vi "Worksheet DOE Audit.vi"(5 "Write Form":bool, 6 "Add?":bool, 7 "Calibration Data":string[][](array[string]), 8 "Low Power\nSwitch":bool, 9 "DOE Data":T1={"Technician"="", "Date"="", "Model"="", "Serial"="", "Total Dry Time(m)"=0.0, "Bone Dry Wt"=0.0, "Initial Wt"=0.0, "Final Wt"=0.0, "Initial Ret"=0.0, "Final Ret"=0.0, "Elect Energy Used"=0.0, "Gas Meter Temp"=0.0, "Gas Meter Pres"=0.0, "Gas Volume"=0.0, "Barometer Temp"=70.0, "Barometer Pres"=0.0, "Gas Corr Fact"=0.0, "Cor Gas Vol"=0.0, "Gas Heat Val"=0.0, "Gas Energy BTU"=0.0, "Gas Energy kwh 4%"=0.0, "Elect Energy kwh 4%"=0.0, "Total  Energy 4%"=0.0, "Gas Vol Init"=0.0, "Gas Vol Fin"=0.0, "Start Time(s)"=0.0, "End Time(s)"=0.0, "Elect Energy Start"=0.0, "Elect Energy End"=0.0, "Per Cycle Efficency"=0.0, "Annual Consumption"=0.0, "Load Cycles"="", "Ambinet Temp"="", "Ambinet RH"="", "Per Cycle Off Mode/Standby Power"=0.0, "Total Energy (Gas + Elect)"=0.0, "Combined Energy Factor"=0.0, "Off Mode Power"=0.0, "Exhaust"="", "Washer Water Temperature ( 60 ± 5°F )"="", "Supply Voltage"="", "Reference Temperature (F)"="", "Reference Pressure (psi)"="", "Standby Power"=0.0}, 10 "2015?":bool) -> (0 "String":string, 1 "2015 array":string[][](array[string]), 2 "DOE Data Out":T1={"Technician"="", "Date"="", "Model"="", "Serial"="", "Total Dry Time(m)"=0.0, "Bone Dry Wt"=0.0, "Initial Wt"=0.0, "Final Wt"=0.0, "Initial Ret"=0.0, "Final Ret"=0.0, "Elect Energy Used"=0.0, "Gas Meter Temp"=0.0, "Gas Meter Pres"=0.0, "Gas Volume"=0.0, "Barometer Temp"=70.0, "Barometer Pres"=0.0, "Gas Corr Fact"=0.0, "Cor Gas Vol"=0.0, "Gas Heat Val"=0.0, "Gas Energy BTU"=0.0, "Gas Energy kwh 4%"=0.0, "Elect Energy kwh 4%"=0.0, "Total  Energy 4%"=0.0, "Gas Vol Init"=0.0, "Gas Vol Fin"=0.0, "Start Time(s)"=0.0, "End Time(s)"=0.0, "Elect Energy Start"=0.0, "Elect Energy End"=0.0, "Per Cycle Efficency"=0.0, "Annual Consumption"=0.0, "Load Cycles"="", "Ambinet Temp"="", "Ambinet RH"="", "Per Cycle Off Mode/Standby Power"=0.0, "Total Energy (Gas + Elect)"=0.0, "Combined Energy Factor"=0.0, "Off Mode Power"=0.0, "Exhaust"="", "Washer Water Temperature ( 60 ± 5°F )"="", "Supply Voltage"="", "Reference Temperature (F)"="", "Reference Pressure (psi)"="", "Standby Power"=0.0})   [LabVIEW 2012]
uses:
  DOE Audit Data.ctl
panel:
  out "Array":string[](array[string])=["tech", "mod", "sn", "loadcy", "dat", "exh", "baro", "wwt", "gm", "sc", "wt5", "gmpt", "ni", "barop", "barot", "rhs", "rhs2", "ts1", "ts2", "gtt", "sca", "tp1", "tp2", "ambt", "ambrh", "gmp", "gmt", "sv", "ghv", "rp", "rt", "bdw", "iw", "fw", "iret", "fr", "tdt", "eeu", "gv", "gcf", "gebtu", "tege", "te4", "om", "sp", "pcomsp", "P", "cef", "ac"]
  out "Column Data":string[](array[string])
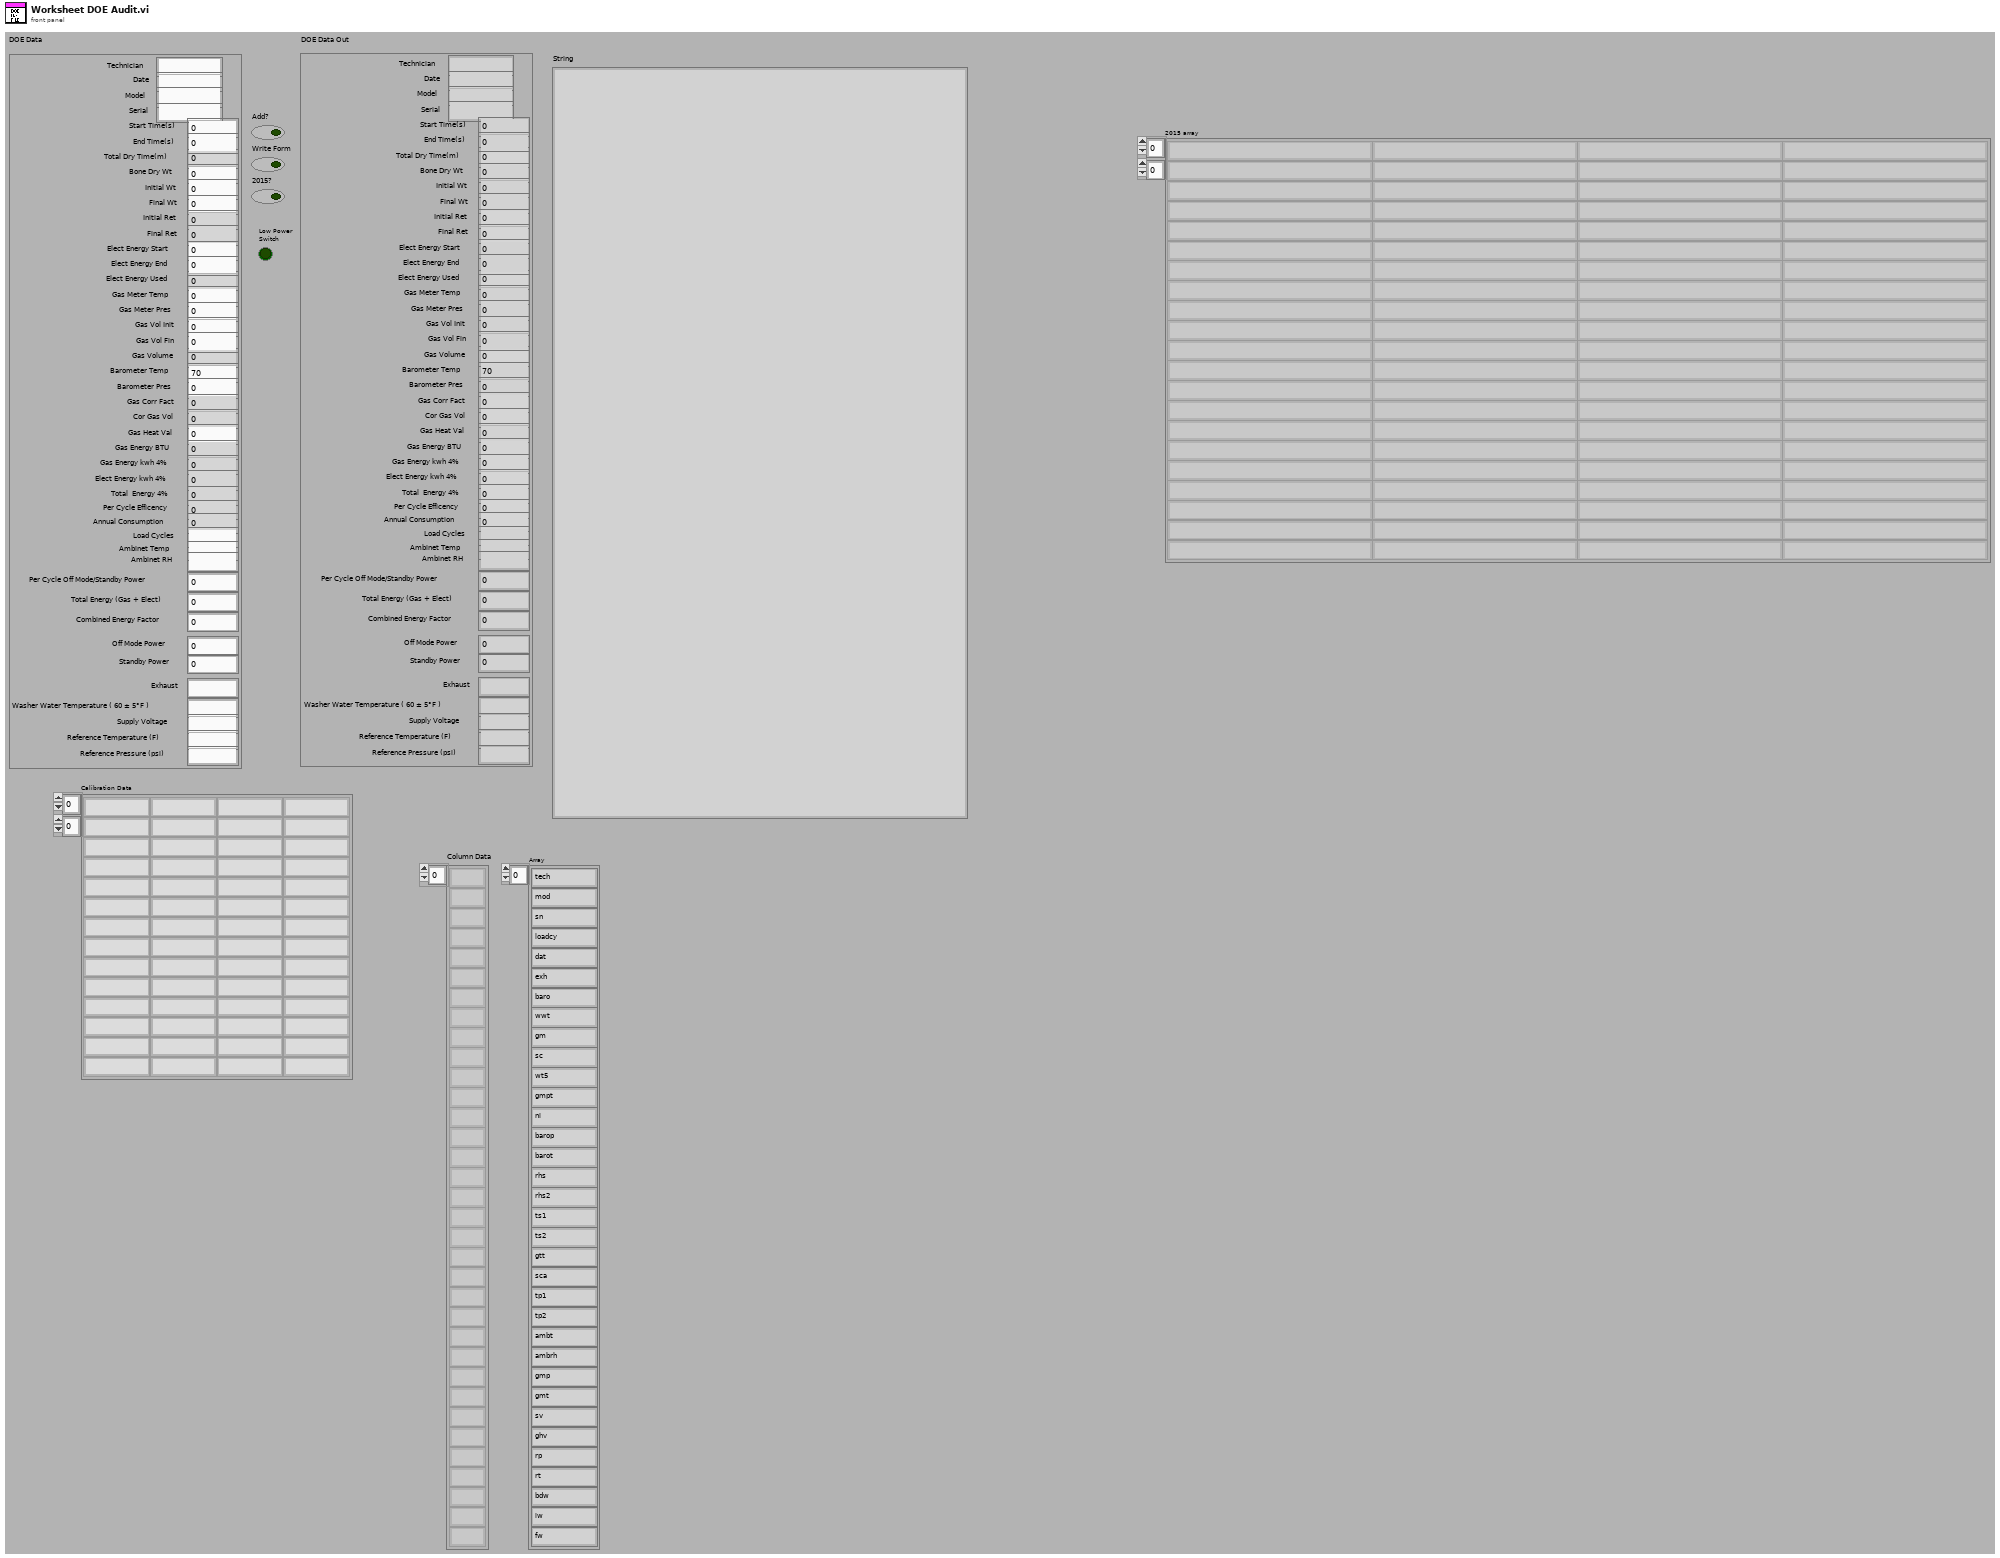
[diagram p1: front panel]
types:
  T1 = typedef "DOE Audit Data.ctl" = cluster{"Technician":string, "Date":string, "Model":string, "Serial":string, "Total Dry Time(m)":dbl, "Bone Dry Wt":dbl, "Initial Wt":dbl, "Final Wt":dbl, "Initial Ret":dbl, "Final Ret":dbl, "Elect Energy Used":dbl, "Gas Meter Temp":dbl, "Gas Meter Pres":dbl, "Gas Volume":dbl, "Barometer Temp":dbl, "Barometer Pres":dbl, "Gas Corr Fact":dbl, "Cor Gas Vol":dbl, "Gas Heat Val":dbl, "Gas Energy BTU":dbl, "Gas Energy kwh 4%":dbl, "Elect Energy kwh 4%":dbl, "Total  Energy 4%":dbl, "Gas Vol Init":dbl, "Gas Vol Fin":dbl, "Start Time(s)":dbl, "End Time(s)":dbl, "Elect Energy Start":dbl, "Elect Energy End":dbl, "Per Cycle Efficency":dbl, "Annual Consumption":dbl, "Load Cycles":string, "Ambinet Temp":string, "Ambinet RH":string, "Per Cycle Off Mode/Standby Power":dbl, "Total Energy (Gas + Elect)":dbl, "Combined Energy Factor":dbl, "Off Mode Power":dbl, "Exhaust":string, "Washer Water Temperature ( 60 ± 5°F )":string, "Supply Voltage":string, "Reference Temperature (F)":string, "Reference Pressure (psi)":string, "Standby Power":dbl}
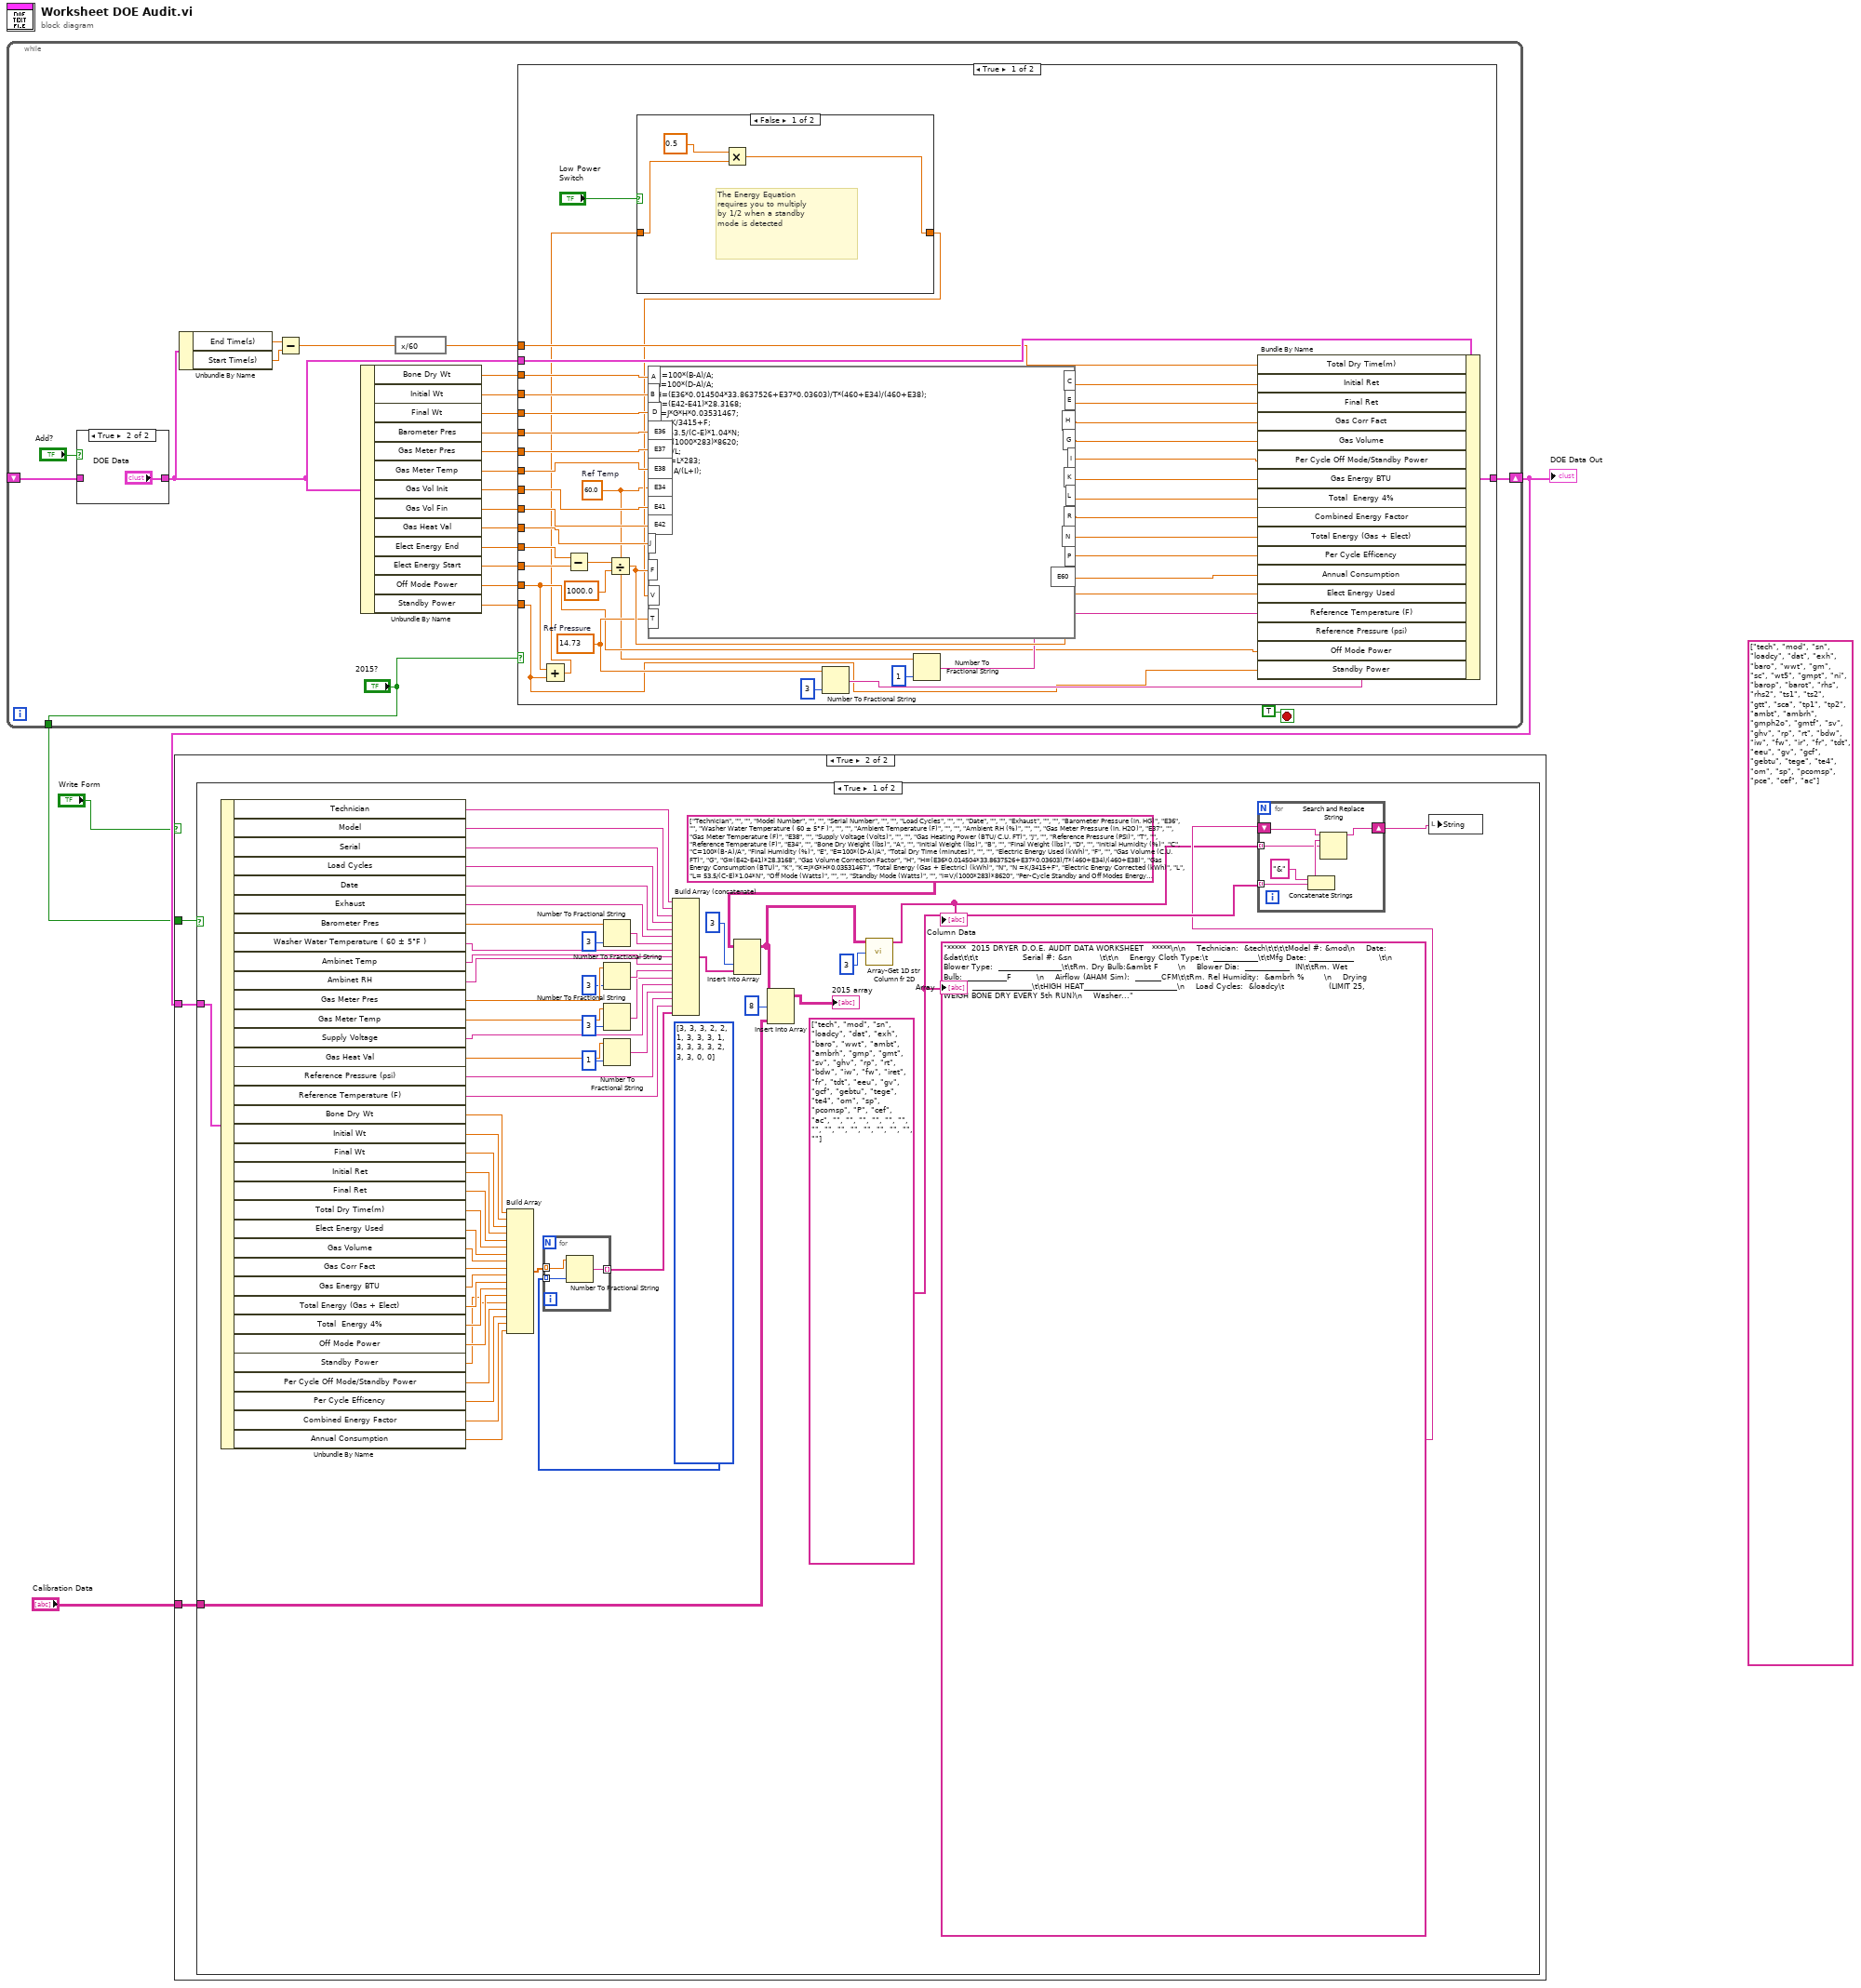
[diagram p0: block diagram]
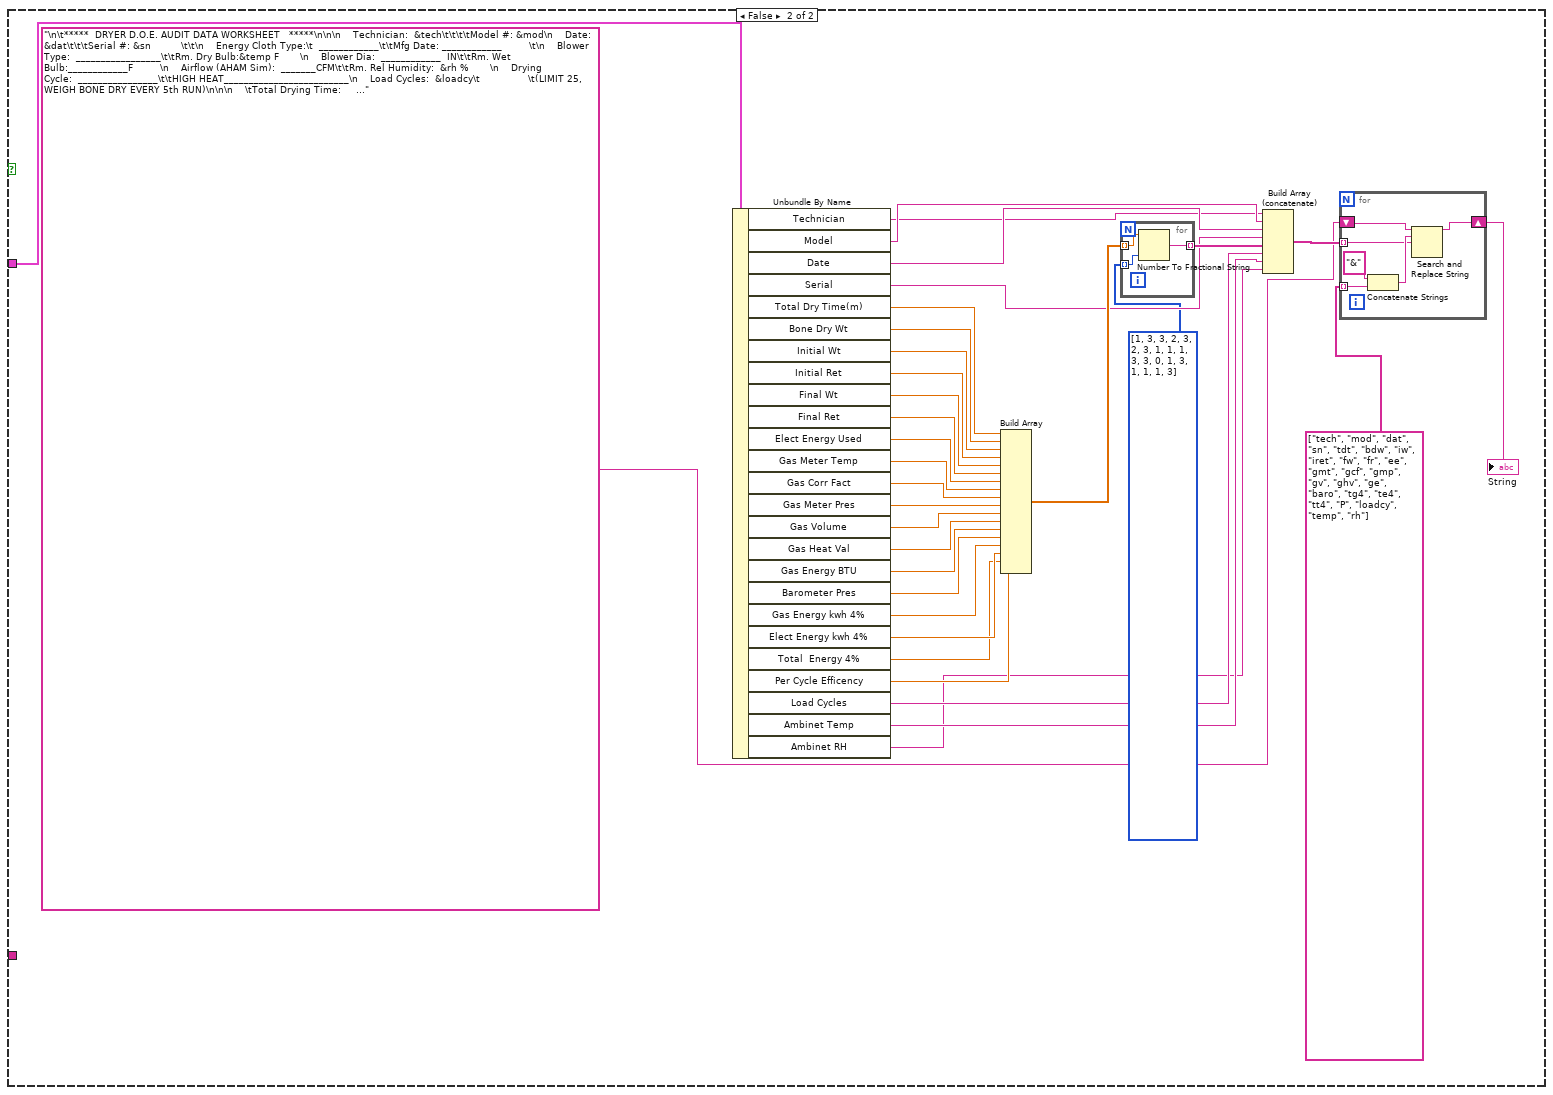
[diagram p3: hidden frame]
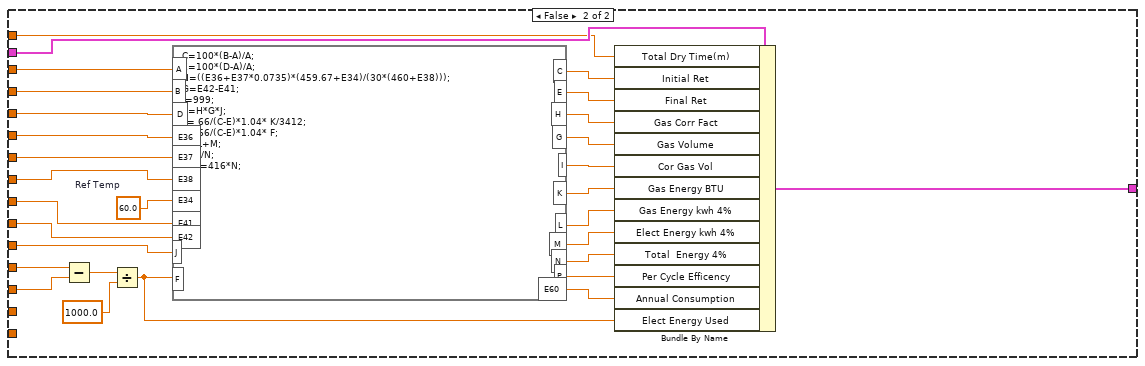
[diagram p5: hidden frame]
diagram:
  (unwired) string[] ["tech", "mod", "sn", "loadcy", "dat", "exh", "baro", "wwt", "gm", "sc", "wt5", "gmpt", "ni", "barop", "barot", "rhs", "rhs2", "ts1", "ts2", "gtt", "sca", "tp1", "tp2", "ambt", "ambrh", "gmph2o", "gmtf", "sv", "ghv", "rp", "rt", "bdw", "iw", "fw", "ir", "fr", "tdt", "eeu", "gv", "gcf", "gebtu", "tege", "te4", "om", "sp", "pcomsp", "pce", "cef", "ac"]
  n1 = while {
    shift-right: [w8] -> w4
    shift-left: _ -> [w26]
    tunnel: ["2015?"] -> w2
    stop <- TRUE stop-if-true
    n2 = case shown="True" "Add?" {
      tunnel: [w100 "DOE Data"] -> w9
      tunnel: w26 -> [w100 _]
      frame False {
      }
      frame True {
      }
    }
    n3 = Unbundle By Name(w9) -> ("End Time(s)"=w24:dbl, "Start Time(s)"=w23:dbl)
    n4 = Subtract(x=w24, y=w23) -> (x-y=w16:dbl)
    n5 = Unbundle By Name(w9) -> ("Bone Dry Wt"=w22:dbl, "Initial Wt"=w21:dbl, "Final Wt"=w20:dbl, "Barometer Pres"=w19:dbl, "Gas Meter Pres"=w18:dbl, "Gas Meter Temp"=w17:dbl, "Gas Vol Init"=w15:dbl, "Gas Vol Fin"=w14:dbl, "Gas Heat Val"=w13:dbl, "Elect Energy End"=w12:dbl, "Elect Energy Start"=w11:dbl, "Off Mode Power"=w10:dbl, "Standby Power"=w5:dbl)
    n6 = expression code="x/60"(w16) -> (w7:dbl)
    n7 = case shown="True" "2015?" {
      tunnel: w22 -> [w66 w99]
      tunnel: w21 -> [w65 w98]
      tunnel: w20 -> [w64 w97]
      tunnel: w19 -> [w63 w95]
      tunnel: w18 -> [w62 w94]
      tunnel: w17 -> [w61 w93]
      tunnel: w15 -> [w60 w92]
      tunnel: w14 -> [w59 w91]
      tunnel: w13 -> [w58 w90]
      tunnel: w12 -> [w57 w89]
      tunnel: w11 -> [w56 w88]
      tunnel: w10 -> [w33 _]
      tunnel: w9 -> [w53 w85]
      tunnel: [w42 w84] -> w8
      tunnel: w7 -> [w52 w83]
      tunnel: w5 -> [w34 _]
      frame True {
        w39 = 14.73  # Ref Pressure
        w28 = 60.0  # Ref Temp
        n8 = Add(x=w33, y=w34) -> (x+y=w30:dbl)
        n9 = Subtract(x=w57, y=w56) -> (x-y=w55:dbl)
        n10 = Divide(x=w55, y=1000.0) -> (x/y=w41:dbl)
        n11 = case shown="False" "Low Power\nSwitch" {
          tunnel: w30 -> [w69 w70]
          tunnel: [w67 w70] -> w29
          frame False {
            # "The Energy Equation \nrequires you to multiply\nby 1/2 when a standby\nmode is detected"
            n12 = Multiply(x=0.5, y=w69) -> (x*y=w67:dbl)
          }
          frame True {
          }
        }
        n13 = formula code="C=100*(B-A)/A;\nE=100*(D-A)/A;\nH=(E36*0.014504*33.8637526+E37*0.03603)/T*(460+E34)/(460+E38);\nG=(E42-E41)*28.3168;\nK=J*G*H*0.03531467;\nN =K/3415+F;\nL= 53.5/(C-E)*1.04*N;\nI=V/(1000*283)*8620;\nP=A/L;\nE60=L*283;\nR = A/(L+I);"("A"=w66, "B"=w65, "D"=w64, "E36"=w63, "E37"=w62, "E34"=w28, "E38"=w61, "E41"=w60, "E42"=w59, "J"=w58, "F"=w41, "V"=w29, "T"=w39) -> ("C"=w51:dbl, "E"=w50:dbl, "H"=w49:dbl, "G"=w48:dbl, "I"=w31:dbl, "K"=w47:dbl, "L"=w46:dbl, "R"=w43:dbl, "N"=w45:dbl, "P"=w44:dbl, "E60"=w37:dbl)
        n14 = Number To Fractional String(number=w39, precision (6)=i16 3) -> (F-format string=w38:string)  [unwired: 2 in]
        n15 = Number To Fractional String(number=w28, precision (6)=i16 1) -> (F-format string=w40:string)  [unwired: 2 in]
        n16 = Bundle By Name(cluster=w53, "Total Dry Time(m)"=w52, "Initial Ret"=w51, "Final Ret"=w50, "Gas Corr Fact"=w49, "Gas Volume"=w48, "Per Cycle Off Mode/Standby Power"=w31, "Gas Energy BTU"=w47, "Total  Energy 4%"=w46, "Combined Energy Factor"=w43, "Total Energy (Gas + Elect)"=w45, "Per Cycle Efficency"=w44, "Annual Consumption"=w37, "Elect Energy Used"=w41, "Reference Temperature (F)"=w40, "Reference Pressure (psi)"=w38, "Off Mode Power"=w33, "Standby Power"=w34) -> (w42:T1)
      }
      frame False {
        w96 = 60.0  # Ref Temp
        n17 = Subtract(x=w89, y=w88) -> (x-y=w87:dbl)
        n18 = Divide(x=w87, y=1000.0) -> (x/y=w71:dbl)
        n19 = formula code="C=100*(B-A)/A;\nE=100*(D-A)/A;\nH=((E36+E37*0.0735)*(459.67+E34)/(30*(460+E38)));\nG=E42-E41;\nI=999;\nK=H*G*J;\nL= 66/(C-E)*1.04* K/3412;\nM=66/(C-E)*1.04* F;\nN=L+M;\nP=A/N;\nE60=416*N;"("A"=w99, "B"=w98, "D"=w97, "E36"=w95, "E37"=w94, "E34"=w96, "E38"=w93, "E41"=w92, "E42"=w91, "J"=w90, "F"=w71) -> ("C"=w82:dbl, "E"=w81:dbl, "H"=w80:dbl, "G"=w79:dbl, "I"=w78:dbl, "K"=w77:dbl, "L"=w76:dbl, "M"=w75:dbl, "N"=w74:dbl, "P"=w73:dbl, "E60"=w72:dbl)
        n20 = Bundle By Name(cluster=w85, "Total Dry Time(m)"=w83, "Initial Ret"=w82, "Final Ret"=w81, "Gas Corr Fact"=w80, "Gas Volume"=w79, "Cor Gas Vol"=w78, "Gas Energy BTU"=w77, "Gas Energy kwh 4%"=w76, "Elect Energy kwh 4%"=w75, "Total  Energy 4%"=w74, "Per Cycle Efficency"=w73, "Annual Consumption"=w72, "Elect Energy Used"=w71) -> (w84:T1)
      }
    }
  }
  "DOE Data Out" <- w4
  n21 = case shown="True" "Write Form" {
    tunnel: w4 -> [_ w104]
    tunnel: w2 -> [_ w103]
    tunnel: "Calibration Data" -> [_ w102]
    frame False {
    }
    frame True {
      n22 = case shown="True" w103 {
        tunnel: w104 -> [w159 w204]
        tunnel: w102 -> [w113 _]
        frame True {
          w111 = string[] ["tech", "mod", "sn", "loadcy", "dat", "exh", "baro", "wwt", "ambt", "ambrh", "gmp", "gmt", "sv", "ghv", "rp", "rt", "bdw", "iw", "fw", "iret", "fr", "tdt", "eeu", "gv", "gcf", "gebtu", "tege", "te4", "om", "sp", "pcomsp", "P", "cef", "ac", "", "", "", "", "", "", "", "", "", "", "", "", "", "", ""]
          n23 = Unbundle By Name(w159) -> ("Technician"=w158:string, "Model"=w157:string, "Serial"=w156:string, "Load Cycles"=w155:string, "Date"=w154:string, "Exhaust"=w153:string, "Barometer Pres"=w152:dbl, "Washer Water Temperature ( 60 ± 5°F )"=w150:string, "Ambinet Temp"=w149:string, "Ambinet RH"=w148:string, "Gas Meter Pres"=w147:dbl, "Gas Meter Temp"=w145:dbl, "Supply Voltage"=w143:string, "Gas Heat Val"=w142:dbl, "Reference Pressure (psi)"=w140:string, "Reference Temperature (F)"=w139:string, "Bone Dry Wt"=w138:dbl, "Initial Wt"=w137:dbl, "Final Wt"=w136:dbl, "Initial Ret"=w135:dbl, "Final Ret"=w134:dbl, "Total Dry Time(m)"=w133:dbl, "Elect Energy Used"=w132:dbl, "Gas Volume"=w131:dbl, "Gas Corr Fact"=w130:dbl, "Gas Energy BTU"=w129:dbl, "Total Energy (Gas + Elect)"=w128:dbl, "Total  Energy 4%"=w127:dbl, "Off Mode Power"=w126:dbl, "Standby Power"=w114:dbl, "Per Cycle Off Mode/Standby Power"=w125:dbl, "Per Cycle Efficency"=w124:dbl, "Combined Energy Factor"=w123:dbl, "Annual Consumption"=w122:dbl)
          n24 = Build Array(w138, w137, w136, w135, w134, w133, w132, w131, w130, w129, w128, w127, w126, w114, w125, w124, w123, w122) -> (w162:dbl[])
          n25 = for {
            tunnel: w162 -> [w169] mode=indexing
            tunnel: [w171] -> w161 mode=indexing
            tunnel: i16[] [3, 3, 3, 2, 2, 1, 3, 3, 3, 1, 3, 3, 3, 3, 2, 3, 3, 0, 0] -> [w170] mode=indexing
            n26 = Number To Fractional String(number=w169, precision (6)=w170) -> (F-format string=w171:string)  [unwired: 2 in]
          }
          n27 = Number To Fractional String(number=w152, precision (6)=i16 3) -> (F-format string=w151:string)  [unwired: 2 in]
          n28 = Number To Fractional String(number=w147, precision (6)=i16 3) -> (F-format string=w146:string)  [unwired: 2 in]
          n29 = Number To Fractional String(number=w145, precision (6)=i16 3) -> (F-format string=w144:string)  [unwired: 2 in]
          n30 = Number To Fractional String(number=w142, precision (6)=i16 1) -> (F-format string=w141:string)  [unwired: 2 in]
          n31 = Build Array (concatenate)(w158, w157, w156, w155, w154, w153, w151, w150, w149, w148, w146, w144, w143, w141, w140, w139, w161) -> (w119:string[])
          n32 = Insert Into Array(array=string[][] [["Technician", "", ""], ["Model Number", "", ""], ["Serial Number", "", ""], ["Load Cycles", "", ""], ["Date", "", ""], ["Exhaust", "", ""], ["Barometer Pressure (in. HG)", "E36", ""], ["Washer Water Temperature ( 60 ± 5°F )", "", ""], ["Ambient Temperature (F)", "", ""], ["Ambient RH (%)", "", ""], ["Gas Meter Pressure (in. H2O)", "E37", ""], ["Gas Meter Temperature (F)", "E38", ""], ["Supply Voltage (Volts)", "", ""], ["Gas Heating Power (BTU/ C.U. FT)", "J", ""], ["Reference Pressure (PSI)", "T", ""], ["Reference Temperature (F)", "E34", ""], ["Bone Dry Weight (lbs)", "A", ""], ["Initial Weight (lbs)", "B", ""], ["Final Weight (lbs)", "D", ""], ["Initial Humidity (%)", "C", "C=100*(B-A)/A"], ["Final Humidity (%)", "E", "E=100*(D-A)/A"], ["Total Dry Time (minutes)", "", ""], ["Electric Energy Used (kWh)", "F", ""], ["Gas Volume (C.U. FT)", "G", "G=(E42-E41)*28.3168"], ["Gas Volume Correction Factor", "H", "H=(E36*0.014504*33.8637526+E37*0.03603)/T*(460+E34)/(460+E38)"], ["Gas Energy Consumption (BTU)", "K", "K=J*G*H*0.03531467"], ["Total Energy (Gas + Electric) (kWh)", "N", "N =K/3415+F"], ["Electric Energy Corrected (kWh)", "L", "L= 53.5/(C-E)*1.04*N"], ["Off Mode (Watts)", "", ""], ["Standby Mode (Watts)", "", "I=V/(1000*283)*8620"], ["Per-Cycle Standby and Off Modes Energy Consumption (kWh)", "I", "P=A/L"], ["Energy Factor (lb/kWh)", "P", "R = A/(L+I)"], ["Combined Energy Factor", "R", "E60=L*283"], ["Annual Energy Consumption (kWh/Year)", "E60", ""], ["", "", ""], ["", "", ""]], index (col)=3 ("disabled index (col)"), new element=w119) -> (w105:string[][])  [unwired: 1 in]
          n33 = Insert Into Array(array=w105, index (row)=8, new element=w113) -> (→"2015 array":string[][])  [unwired: 1 in]
          n34 = call "Array-Get 1D str Column fr 2D.vi"("2D Array Data"=w105, "column index"=3) -> ("Column Data"=w106:string[])  [unwired: 13 in]
          "Column Data" <- w106
          n35 = for {
            tunnel: w111 -> [w167] mode=indexing
            tunnel: w106 -> [w164] mode=indexing
            shift-right: [w163] -> w109
            shift-left: "*****  2015 DRYER D.O.E. AUDIT DATA WORKSHEET   *****\n\n    Technician:  &tech\t\t\t\tModel #: &mod\n    Date:  &dat\t\t\t                Serial #: &sn          \t\t\n    Energy Cloth Type:\t  ____________\t\tMfg Date: ____________         \t\n    Blower Type:  _________________\t\tRm. Dry Bulb:&ambt F       \n    Blower Dia:  ____________  IN\t\tRm. Wet Bulb:____________F         \n    Airflow (AHAM Sim):  _______CFM\t\tRm. Rel Humidity:  &ambrh %       \n    Drying Cycle:  ________________\t\tHIGH HEAT_________________________\n    Load Cycles:  &loadcy\t                (LIMIT 25, WEIGH BONE DRY EVERY 5th RUN)\n    Washer Water Temperature ( 60 ± 5°F ): &wwt\n    Exhaust Type: &exh\n    Equipment Calibration: Reference Spreadsheet File\n\n    \tTotal Drying Time:     &tdt  min\n(A) \tBone Dry Weight:       &bdw lb\t\t\t(ALL WEIGHTS FROM REF SCALE)\n(B) \tInitial Wt. Wet Load:  &iw  lb\t\t(C) Initial Ret. 100*(B-A)/A:  &iret %\n(D) \tFinal Wt. Dried Load:  &fw  lb\t\t(E) Final Ret.   100*(D-A)/A:  &fr %\n\nELECTRICAL ENERGY:\n\n(F) Electrical Energy Used:  &eeu  kwh\n\nGAS ENERGY:\n\n\tGas Meter Temp:   &gmt F\t   (H) Gas Corr. Factor:     &gcf  ++ \n\tGas Meter Press:  &gmp in H20      (J) Gas Heating Value:    &ghv  BTU/CUFT           \n(G) Metered Gas Vol:      &gv Liters (K) Gas Energy (G*H*J*0.0353):     &gebtu BTU\t     \n           \nBarometer Press:  &baro in HG\t           Supply Voltage: &sv\t\n\nReference Pressure: &rp                    Reference Temperature: &rt\n\n++ From PC program per US Bureau of Stds, C417,1938\n \n(N) Total Energy (Gas + Electric) (kWh): &tege\n    [(K/3415)+F]\n\n(L) Per cycle Total Electric Energy Consumption adjusted to 4%:  &te4 KWH/CYCLE\n    ([53.5/(C-E)]*1.04*N)\n\n(I) Per Cycle Off Mode/Standby Mode Power: &pcomsp\n    [V/(1000*283)*8620] \n\n(V) Standby Mode Power: &sp Watts\n    Off Mode Power: &om Watts \n         Off Mode > 0 & Standby Mode > 0: [0.5*(Off Mode+Standby Mode)]\n         Off Mode > 0 & Standby Mode = 0: [(Off Mode+Standby Mode)]\n\n(E60) Annual Consumption: [(L*283)]  &ac kwh\n\n(R) Combined Energy Factor: [A/(L+I)] &cef\n\n***********************************************************\n   * (P) Per Cycle Energy Efficiency (A/L): &P\n***********************************************************" -> [w168]
            n36 = Concatenate Strings("&" ("string"), w167) -> (w165:string)
            n37 = Search and Replace String(input string=w168, search string=w165, replace string=w164) -> (result string=w163:string)  [unwired: 5 in, 3 out]
          }
          n38 = local write "String"(w109) -> ()
          "Array" <- w111
        }
        frame False {
          n39 = Unbundle By Name(w204) -> ("Technician"=w181:string, "Model"=w182:string, "Date"=w183:string, "Serial"=w184:string, "Total Dry Time(m)"=w203:dbl, "Bone Dry Wt"=w202:dbl, "Initial Wt"=w201:dbl, "Initial Ret"=w200:dbl, "Final Wt"=w199:dbl, "Final Ret"=w198:dbl, "Elect Energy Used"=w197:dbl, "Gas Meter Temp"=w196:dbl, "Gas Corr Fact"=w195:dbl, "Gas Meter Pres"=w194:dbl, "Gas Volume"=w193:dbl, "Gas Heat Val"=w192:dbl, "Gas Energy BTU"=w191:dbl, "Barometer Pres"=w190:dbl, "Gas Energy kwh 4%"=w189:dbl, "Elect Energy kwh 4%"=w188:dbl, "Total  Energy 4%"=w173:dbl, "Per Cycle Efficency"=w187:dbl, "Load Cycles"=w178:string, "Ambinet Temp"=w176:string, "Ambinet RH"=w175:string)
          n40 = Build Array(w203, w202, w201, w200, w199, w198, w197, w196, w195, w194, w193, w192, w191, w190, w189, w188, w173, w187) -> (w186:dbl[])
          n41 = for {
            tunnel: w186 -> [w207] mode=indexing
            tunnel: [w206] -> w185 mode=indexing
            tunnel: i16[] [1, 3, 3, 2, 3, 2, 3, 1, 1, 1, 3, 3, 0, 1, 3, 1, 1, 1, 3] -> [w205] mode=indexing
            n42 = Number To Fractional String(number=w207, precision (6)=w205) -> (F-format string=w206:string)  [unwired: 2 in]
          }
          n43 = Build Array (concatenate)(w181, w182, w183, w184, w185, w178, w176, w175) -> (w179:string[])
          n44 = for {
            tunnel: string[] ["tech", "mod", "dat", "sn", "tdt", "bdw", "iw", "iret", "fw", "fr", "ee", "gmt", "gcf", "gmp", "gv", "ghv", "ge", "baro", "tg4", "te4", "tt4", "P", "loadcy", "temp", "rh"] -> [w212] mode=indexing
            tunnel: w179 -> [w209] mode=indexing
            shift-right: [w208] -> w172
            shift-left: "\n\t*****  DRYER D.O.E. AUDIT DATA WORKSHEET   *****\n\n\n    Technician:  &tech\t\t\t\tModel #: &mod\n    Date:  &dat\t\t\tSerial #: &sn          \t\t\n    Energy Cloth Type:\t  ____________\t\tMfg Date: ____________         \t\n    Blower Type:  _________________\t\tRm. Dry Bulb:&temp F       \n    Blower Dia:  ____________  IN\t\tRm. Wet Bulb:____________F         \n    Airflow (AHAM Sim):  _______CFM\t\tRm. Rel Humidity:  &rh %       \n    Drying Cycle:  ________________\t\tHIGH HEAT_________________________\n    Load Cycles:  &loadcy\t                \t(LIMIT 25, WEIGH BONE DRY EVERY 5th RUN)\n\n\n    \tTotal Drying Time:     &tdt  min\n(A) \tBone Dry Weight:       &bdw lb\t\t\t(ALL WEIGHTS FROM REF SCALE)\n(B) \tInitial Wt. Wet Load:  &iw  lb\t\t(C) Initial Ret. [(B-A)/A]:  &iret %\n(D) \tFinal Wt. Dried Load:  &fw  lb\t\t(E) Final Ret.   [(D-A)/A]:  &fr %\n\nELECTRICAL ENERGY:\n\n(F) Electrical Energy Used:  &ee  kwh\n\nGAS ENERGY:\n\n\tGas Meter Temp:   &gmt F\t        \t(H) Gas Corr. Factor:     &gcf  ++ \n\tGas Meter Press:  &gmp in H20           \n(G) Metered Gas Vol:      &gv CU FT\t\t(J) Gas Heating Value:    &ghv  BTU/CUFT\n\t                                        (K) Gas Energy (G*H*J):     &ge BTU\n\tBarometer Press:  &baro in HG\t\t\n\n++ From PC program per US Bureau of Stds, C417,1938 \n\n(M) Per cycle Total Electric Energy Consumption adjusted to 4%:  &te4 KWH/CYCLE\n([66/(C-E)]*1.04*F)\n\n(N) Per cycle Total Gas Energy Consumption adjusted to 4%:  &tg4 KWH/CYCLE\n([66/(C-E)]*1.04*K)/3412\n\n(O) Total Energy Used in kwh (M+N):  &tt4 kwh\n***********************************************************\n   * (P) Per Cycle Energy Efficiency (A/O): &P\n***********************************************************\n" -> [w213]
            n45 = Concatenate Strings("&" ("string"), w212) -> (w210:string)
            n46 = Search and Replace String(input string=w213, search string=w210, replace string=w209) -> (result string=w208:string)  [unwired: 5 in, 3 out]
          }
          "String" <- w172
        }
      }
    }
  }
